vi "h5_stats.vi"(6 "Attributes":variant, 7 "TYPE":string="STATS_0", 8 "error in (no error)":errorcluster, 9 "info":T1, 10 "SQUID":string="1", 11 "H5":path[](array[path])=[path "D:/Data/2015/08/19/20150819_190813/20150819_190813.h5"]) -> (0 "error out":errorcluster, 2 "Exists":bool)   [LabVIEW 2013]
uses:
  statistics.ctl
  <vilib>/addons/h5labview2/file/H5Fmode.ctl
  <vilib>/addons/h5labview2/base/lib_path.vi
  <vilib>/addons/h5labview2/base/H5Equery.vi
  <vilib>/addons/h5labview2/dataset/H5Dwrite.llb/H5Dwrite.xnode
  <vilib>/addons/h5labview2/base/hid_t.ctl
  <vilib>/addons/h5labview2/file/H5F.lvlib
  <vilib>/addons/h5labview2/dataset/H5D.lvlib
  <vilib>/addons/h5labview2/group/H5G.lvlib
  <vilib>/addons/h5labview2/space/H5S.lvlib
  <vilib>/addons/h5labview2/attrib/H5A.lvlib
panel:
  out "error out 2":errorcluster
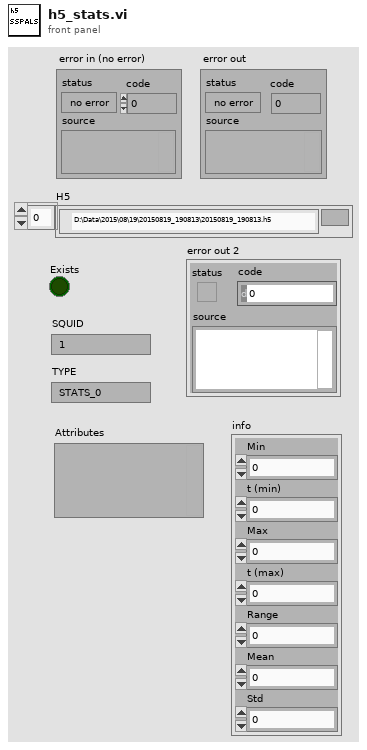
[diagram p1: front panel]
types:
  T1 = typedef "statistics.ctl" = cluster{"Min":dbl, "t (min)":dbl, "Max":dbl, "t (max)":dbl, "Range":dbl, "Mean":dbl, "Std":dbl}
  T2 = typedef "Semaphore RefNum" = refnum<k1>
  T3 = typedef "H5F.lvlib/H5Fmode.ctl" = enum16{"read-only", "read-write", "overwrite", "create new", "open or create"}
  T4 = typedef "hid_t.ctl" = i32
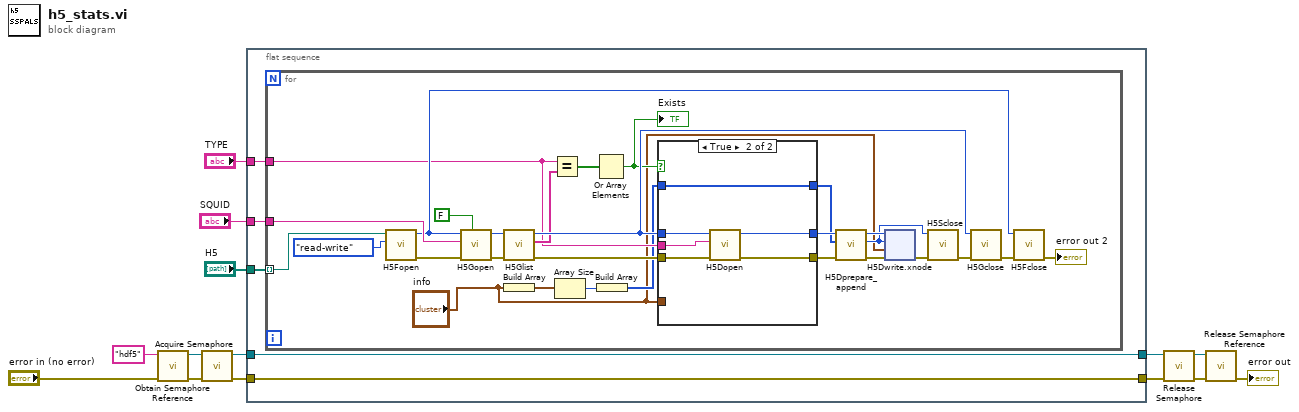
[diagram p0: block diagram]
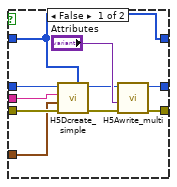
[diagram p2: hidden frame]
diagram:
  n1 = call <vilib>:"Obtain Semaphore Reference.vi"("error in (no error)"="error in (no error)", "name (unnamed)"="hdf5") -> ("error out"=w13:errorcluster, "semaphore"=w14:T2)  [unwired: 3 in, 1 out]
  n2 = call <vilib>:"Acquire Semaphore.vi"("error in (no error)"=w13, "semaphore"=w14) -> ("error out"=w7:errorcluster, "semaphore out"=w6:T2)  [unwired: 3 in, 1 out]
  n3 = flat-sequence {
    tunnel: [w19] -> w8
    tunnel: w7 -> [w19]
    tunnel: w6 -> [w18]
    tunnel: [w18] -> w5
    tunnel: "H5" -> [w17]
    tunnel: "SQUID" -> [w16]
    tunnel: "TYPE" -> [w15]
    frame #0 {
      n4 = for {
        tunnel: w17 -> [w34] mode=indexing
        tunnel: w16 -> [w35]
        tunnel: w15 -> [w26]
        n5 = call <vilib>:"H5Fopen.vi"("mode (read-only)"=H5Fmode."read-write", "path"=w34) -> ("error out"=w33:errorcluster, "ref out"=w32:T4)  [unwired: 8 in]
        n6 = call <vilib>:"H5Gopen.vi"("create? (F)"=FALSE, "error in (no error)"=w33, "name"=w35, "ref in"=w32) -> ("error out"=w30:errorcluster, "group out"=w31:T4)  [unwired: 6 in]
        n7 = call <vilib>:"H5Glist.vi"("error in (no error)"=w30, "ref in"=w31) -> ("error out"=w29:errorcluster, "names"=w27:string[], "ref out"=w28:T4)  [unwired: 6 in, 1 out]
        n8 = Build Array("info") -> (w23:T1[])
        n9 = Equal?(x=w26, y=w27) -> (x = y?=w25:bool[])
        n10 = Array Size(array=w23) -> (size(s)=w22:i32)
        n11 = Or Array Elements(Boolean array=w25) -> (logical OR=w24:bool)
        "Exists" <- w24
        n12 = Build Array(w22) -> (w21:i32[])
        n13 = case shown="True" w24 {
          tunnel: w29 -> [w75 w80]
          tunnel: w28 -> [w74 w77]
          tunnel: w26 -> [w73 w78]
          tunnel: [w70 w79] -> w46
          tunnel: [w71 w76] -> w45
          tunnel: w21 -> [w67 w81]
          tunnel: [w67 w81] -> w42
          tunnel: "info" -> [w66 _]
          frame False {
            n14 = call <vilib>:"H5Dcreate_simple.vi"("chunk size"=w67, "error in (no error)"=w75, "type in"=w66, "name"=w73, "ref in"=w74) -> ("error out"=w69:errorcluster, "dset out"=w68:T4)  [unwired: 5 in]
            n15 = call <vilib>:"H5Awrite_multi.vi"("error in (no error)"=w69, "variant in"="Attributes", "ref in"=w68) -> ("error out"=w70:errorcluster, "ref out"=w71:T4)  [unwired: 7 in]
          }
          frame True {
            n16 = call <vilib>:"H5Dopen.vi"("error in (no error)"=w80, "name"=w78, "loc in"=w77) -> ("error out"=w79:errorcluster, "dset out"=w76:T4)  [unwired: 7 in]
          }
        }
        n17 = call <vilib>:"H5Dprepare_append.vi"("error in (no error)"=w46, "append dims"=w42, "dset in"=w45) -> ("error out"=w44:errorcluster, "space out"=w40:T4, "dset out"=w41:T4)  [unwired: 6 in]
        n18 = xnode "H5Dwrite.xnode"("error in (no error)"=w44, "data"="info", "file space"=w40, "ref in"=w41) -> ("error out"=w43:errorcluster)  [unwired: 3 in, 2 out]
        n19 = call <vilib>:"H5Sclose.vi"("error in (no error)"=w43, "space in"=w40) -> ("error out"=w38:errorcluster)  [unwired: 9 in]
        n20 = call <vilib>:"H5Gclose.vi"("error in (no error)"=w38, "group in"=w28) -> ("error out"=w36:errorcluster)  [unwired: 9 in]
        n21 = call <vilib>:"H5Fclose.vi"("error in (no error)"=w36, "ref"=w32) -> ("error out"=→"error out 2":errorcluster)  [unwired: 9 in]
      }
    }
  }
  n22 = call <vilib>:"Release Semaphore.vi"("error in (no error)"=w8, "semaphore"=w5) -> ("error out"=w9:errorcluster, "semaphore out"=w10:T2)  [unwired: 4 in]
  n23 = call <vilib>:"Release Semaphore Reference.vi"("error in (no error)"=w9, "semaphore"=w10) -> ("error out"=→"error out":errorcluster)  [unwired: 8 in, 1 out]
